vi "SparkMAXPositionToDegrees.vi"(4 "Sensor Position":dbl) -> (1 "degrees":dbl)   [LabVIEW 2019]
panel:
  in  "constant":dbl=0.087890625 format="%#_13g"
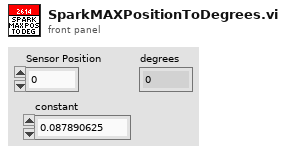
[diagram p1: front panel]
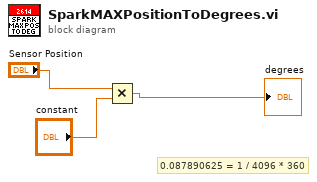
[diagram p0: block diagram]
diagram:
  # "0.087890625 = 1 / 4096 * 360"
  n1 = Multiply(x="Sensor Position", y="constant") -> (x*y=→"degrees":dbl)
